vi "Display.vi"(6 "test fail message":string="Test failed. Failure time: %s", 7 "test pass message":string="Test passed", 8 "error in":errorcluster, 11 "Test Results":refnum<class "Test Results Base Class.lvclass">) -> (0 "error out":errorcluster)   [LabVIEW 2020, in "Test Results Base Class.lvclass"]
doc: "This VI displays a dialog that indicates the test results."
uses:
  Test Results Base Class.lvclass
  Test Results Base Class.lvclass/Test Results Base Class.ctl
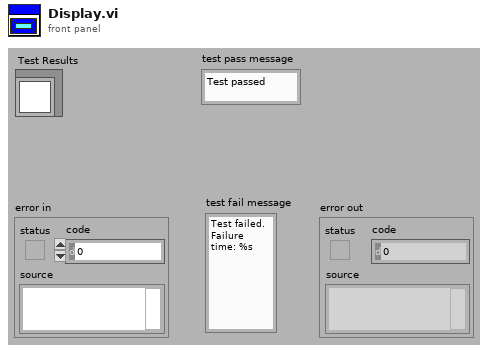
[diagram p1: front panel]
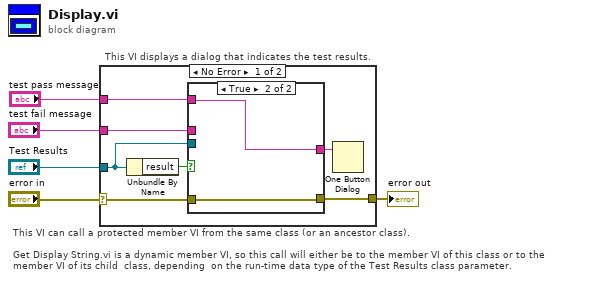
[diagram p0: block diagram]
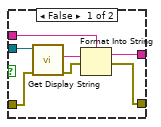
[diagram p2: hidden frame]
diagram:
  # "This VI can call a protected member VI from the same class (or an ancestor class).\n\nGet Display String.vi is a dynamic member VI, so this call will either be to the member VI of this class or to the member VI of its child  class, depending  on the run-time data type of the Test Results class parameter."
  # "This VI displays a dialog that indicates the test results."
  n1 = case shown="No Error" "error in" {
    selector: "error in" -> [w11 w22]
    tunnel: "Test Results" -> [w6 _]
    tunnel: [w9 w22] -> w3
    tunnel: "test fail message" -> [w8 _]
    tunnel: "test pass message" -> [w7 _]
    frame No Error {
      n2 = Unbundle By Name(w6) -> ("result"=w12:bool)
      n3 = case shown="True" w12 {
        tunnel: w11 -> [w14 w21]
        tunnel: [w19 w20] -> w10
        tunnel: [w18 w21] -> w9
        tunnel: w8 -> [w17 _]
        tunnel: w7 -> [_ w20]
        tunnel: w6 -> [w15 _]
        frame False {
          n4 = call-dynamic "Get Display String.vi"("error in"=w14, "test\nresults in"=w15) -> ("error out"=w13:errorcluster, "display string"=w16:string)  [unwired: 7 in, 1 out]
          n5 = Format Into String(format string=w17, error in=w13, w16) -> (resulting string=w19:string, error out=w18:errorcluster)  [unwired: 1 in]
        }
        frame True {
        }
      }
      n6 = One Button Dialog(message=w10) -> ()  [unwired: 1 in, 1 out]
    }
    frame Error {
    }
  }
  "error out" <- w3
